vi "Validate Search Params.vi"(11 "Search Params In":T1) -> (1 "Valid?":bool, 2 "Search Validation Failure":T5, 3 "Search Params":T1)   [LabVIEW 2016, in "Better Search.lvlib" / "BetterSearch.lvclass"]
uses:
  BetterSearch.lvclass
  Search Validation Failure.ctl
  Data Types/Search Type.ctl
  Better Search.lvlib
  Data Types/Search Scope.ctl
  Data Types/Scope Options.ctl
  Data Types/Search Params.ctl
panel:
  # "Exclude"
  # "Exclude"
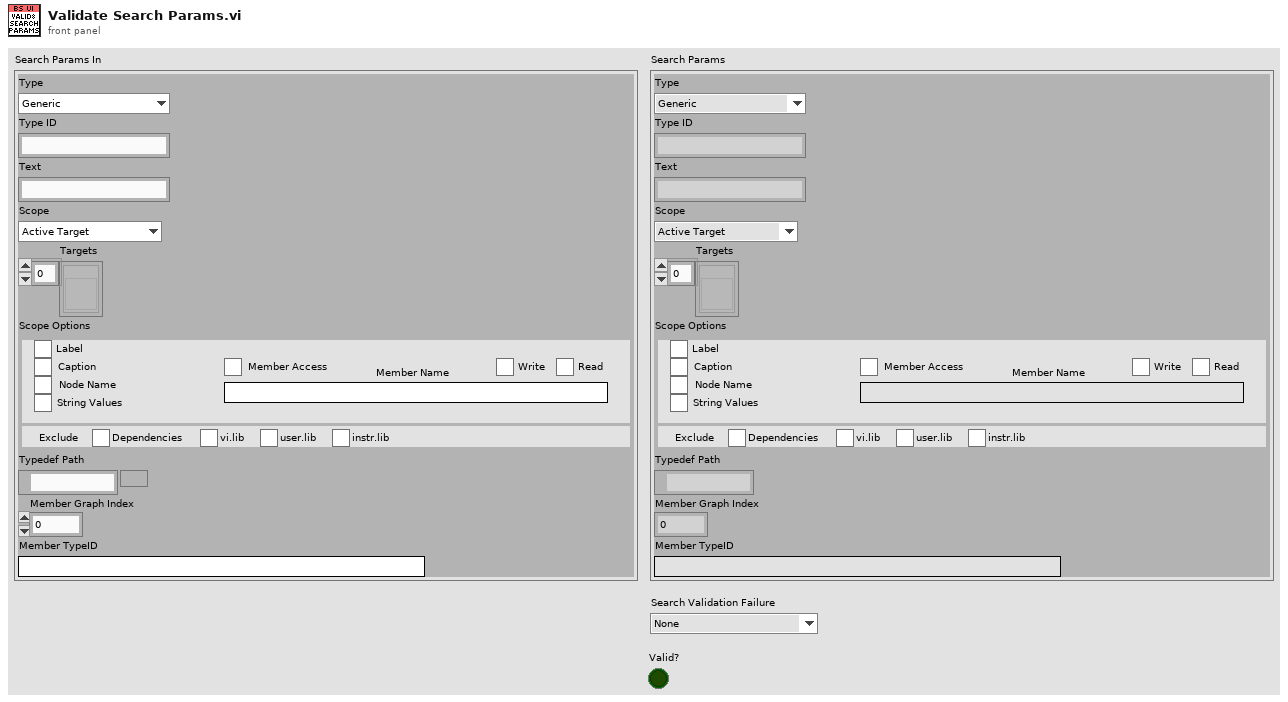
[diagram p1: front panel]
types:
  T1 = typedef "Better Search.lvlib/Search Params.ctl" = cluster{"Type":T2, "Type ID":string, "Text":string, "Scope":T3, "Targets":refnum<vi>[], "Scope Options":T4, "Typedef Path":path, "Member Graph Index":i32, "Member TypeID":string}
  T2 = typedef "Better Search.lvlib/Search Type.ctl" = enum16{"Generic", "Text", "Data Type", "VI", "Node"}
  T3 = typedef "Better Search.lvlib/Search Scope.ctl" = enum16{"Active Target", "Active Project", "Specific Targets", "Active VI", "Active Hierarchy"}
  T4 = typedef "Better Search.lvlib/Scope Options.ctl" = cluster{"Include Labels":bool, "Include Captions":bool, "Include Node Name":bool, "Member Access":bool, "Member Read":bool, "Member Write":bool, "Member Name":string, "String Value":bool, "Dependencies":bool, "vi.lib":bool, "user.lib":bool, "instr.lib":bool}
  T5 = typedef "Better Search.lvlib/BetterSearch.lvclass/Search Validation Failure.ctl" = enum16{"None", "Empty Text"}
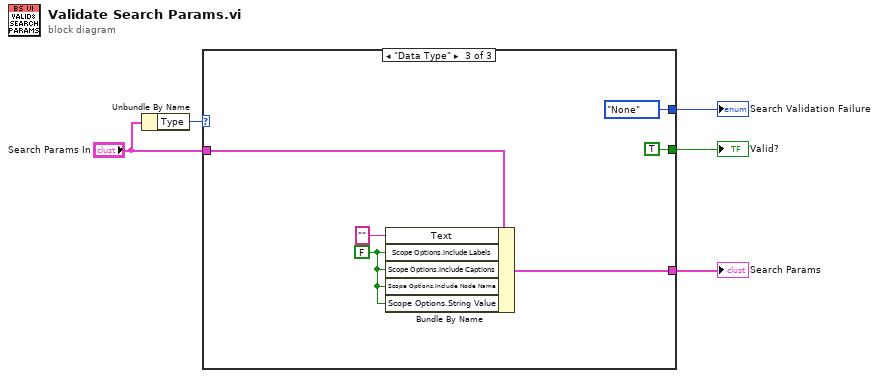
[diagram p0: block diagram]
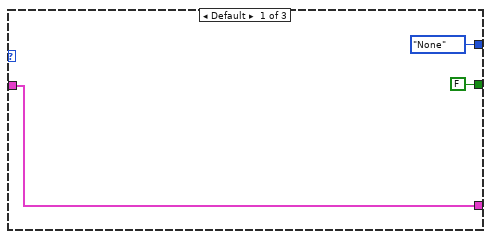
[diagram p2: hidden frame]
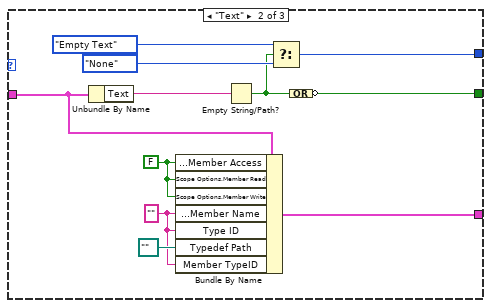
[diagram p3: hidden frame]
diagram:
  n1 = Unbundle By Name("Search Params In") -> ("Type"=w5:T2)
  n2 = case shown="\"Data Type\"" w5 {
    tunnel: "Search Params In" -> [w8 w13 w23]
    tunnel: [FALSE w18 TRUE] -> w3
    tunnel: [Search_Validation_Failure."None" ("Search Validation Failure") w14 Search_Validation_Failure."None" ("Search Validation Failure")] -> w2
    tunnel: [w8 w11 w20] -> w1
    frame Default {
    }
    frame "Text" {
      w9 = "" ("Scope Options.Member Name")
      w12 = FALSE ("Scope Options.Member Access")
      n3 = Unbundle By Name(w13) -> ("Text"=w19:string)
      n4 = Bundle By Name(cluster=w13, "Scope Options.Member Access"=w12, "Scope Options.Member Read"=w12, "Scope Options.Member Write"=w12, "Scope Options.Member Name"=w9, "Type ID"=w9, "Typedef Path"=path "", "Member TypeID"=w9) -> (w11:T1)
      n5 = Empty String/Path?(string/path=w19) -> (empty?=w15:bool)
      n6 = Select(t=Search_Validation_Failure."Empty Text" ("Search Validation Failure"), s=w15, f=Search_Validation_Failure."None" ("Search Validation Failure")) -> (s? t:f=w14:T5)
      n7 = Compound Arithmetic op=OR(w15) -> (invert w18:bool)
    }
    frame "Data Type" {
      w21 = FALSE ("Scope Options.Include Labels")
      n8 = Bundle By Name(cluster=w23, "Text"="", "Scope Options.Include Labels"=w21, "Scope Options.Include Captions"=w21, "Scope Options.Include Node Name"=w21, "Scope Options.String Value"=w21) -> (w20:T1)
    }
  }
  "Valid?" <- w3
  "Search Validation Failure" <- w2
  "Search Params" <- w1
